vi "Unpack for gRPC.vi"(8 "error in":errorcluster, 9 "configuration / results":enum16{"Configuration", "Results"}(ring), 10 "any":T1, 11 "measurement customizations in":refnum<class "Measurement Plugin.lvclass">) -> (0 "error out":errorcluster, 2 "data value":variant, 3 "measurement customizations out":refnum<class "Measurement Plugin.lvclass">)   [LabVIEW 2024, in "Averaged - Broadband.lvlib" / "Measurement Plugin.lvclass"]
uses:
  Measurement Plugin.lvclass
  <vilib>/gRPC/LabVIEW gRPC Library/Shared/Any.ctl
  Measurement Configuration.ctl
  Measurement Results.ctl
  <vilib>/gRPC/Generated APIs/ni/protobuf/types/RPC Messages/ni_protobuf_types_DoubleXYData.ctl
  a521b266-ce99-437c-923d-067dcf1e07fd.vi
  3ecd018e-d556-4cbc-bc60-c4ba57204520.vi
  <vilib>/gRPC/LabVIEW gRPC Library/Server API/Translate Protobuf Error.vi
  <vilib>/AdvancedString/1D String Array to Delimited String.vi
  <vilib>/gRPC/LabVIEW gRPC Library/Server API/Server/Get Server DLL Path.vi
  Measurement Plugin.lvclass/Measurement Plugin.ctl
  Averaged - Broadband.lvlib
  <vilib>/gRPC/Generated APIs/ni/protobuf/types/ni.protobuf.types.lvlib
  <vilib>/Plug-In SDKs/Measurements/Measurement Plugin Service/Measurement Plugin Service.lvclass
  C:/Program Files/National Instruments/LabVIEW 2024/vi.lib/Plug-In SDKs/Measurements/Measurement Plugin Service/Measurement Plugin Service.lvclass
  C:/Git/dsa/source/FRF Stim-Resp/Averaged - Broadband/Advanced/Measurement Plugin.lvclass
  <vilib>/gRPC/LabVIEW gRPC Library/grpc-lvsupport-release.lvlib
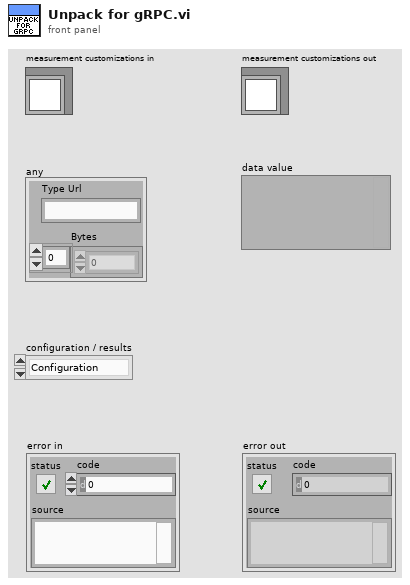
[diagram p1: front panel]
types:
  T1 = typedef "grpc-lvsupport-release.lvlib/Any.ctl" = cluster{"Type Url":string, "Bytes":u8[]}
  T2 = typedef "grpc-lvsupport-release.lvlib/grpcId.ctl" = u64
  T3 = typedef "Averaged - Broadband.lvlib/Measurement Configuration.ctl" = cluster{"double array in":dbl[], "double in":dbl, "U32 array in":u32[], "U32 in":u32, "U64 array in":u64[], "U64 in":u64, "I32 array in":i32[], "I32 in":i32, "I64 array in":i64[], "I64 in":i64, "bool in":bool, "string in":string, "u32 color ring in":u32, "u32 animal enum in":enum32{"Rabbit", "Gopher", "Badger"}}
  T4 = typedef "Averaged - Broadband.lvlib/Measurement Results.ctl" = cluster{"xy data out":T5, "double array out":dbl[], "double out":dbl, "U32 array out":u32[], "U32 out":u32, "U64 array out":u64[], "U64 out":u64, "I32 array out":i32[], "I32 out":i32, "I64 array out":i64[], "I64 out":i64, "bool out":bool, "string out":string, "u32 color ring out":u32, "u32 animal enum out":enum32{"Rabbit", "Gopher", "Badger"}}
  T5 = typedef "ni.protobuf.types.lvlib/ni_protobuf_types_DoubleXYData.ctl" = cluster{"x_data":dbl[], "y_data":dbl[]}
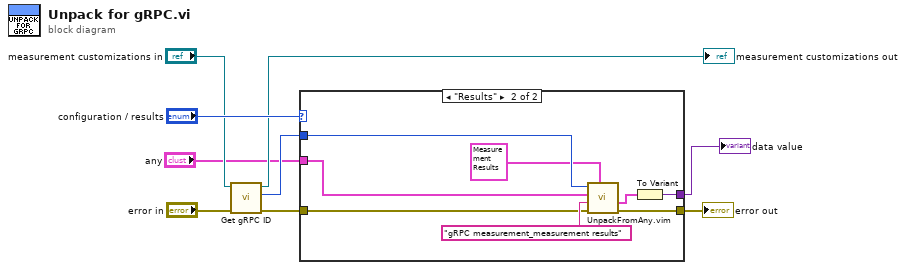
[diagram p0: block diagram]
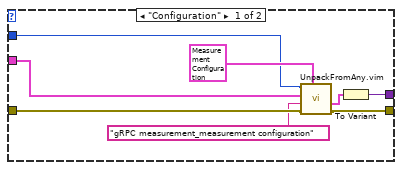
[diagram p2: hidden frame]
diagram:
  n1 = call <vilib>:"Get gRPC ID.vi"("error in"="error in", "measurement plugin service in"="measurement customizations in") -> ("error out"=w6:errorcluster, "gRPC ID"=w3:T2, "measurement plugin service out"=→"measurement customizations out":refnum<class "Measurement Plugin.lvclass">)  [unwired: 7 in]
  n2 = case shown="\"Results\"" "configuration / results" {
    tunnel: w6 -> [w15 w19]
    tunnel: "any" -> [w10 w18]
    tunnel: w3 -> [w12 w22]
    tunnel: [w16 w23] -> w9
    tunnel: [w17 w25] -> w1
    frame "Configuration" {
      n3 = call "UnpackFromAny.vim"("Data Type"=T3 {"double array in"=[], "double in"=1.2, "U32 array in"=[32, 33], "U32 in"=32, "U64 array in"=[64, 65], "U64 in"=64, "I32 array in"=[-32, -33], "I32 in"=-32, "I64 array in"=[-64, -65], "I64 in"=-64, "bool in"=TRUE, "string in"="Lorem ipsum dolor sit", "u32 color ring in"=1, "u32 animal enum in"=enum."Gopher"} ("Measurement Configuration"), "error in"=w15, "Message Type"="gRPC measurement_measurement configuration", "Any"=w10, "gRPCid in"=w12) -> ("error out"=w16:errorcluster, "Unpacked Value"=w14:T3)  [unwired: 4 in, 1 out]
      n4 = To Variant(anything=w14) -> (Variant=w17:variant)
    }
    frame "Results" {
      n5 = call "UnpackFromAny.vim"("Data Type"=T4 {"xy data out"={"x_data"=[], "y_data"=[]}, "double array out"=[], "double out"=0.0, "U32 array out"=[0], "U32 out"=0, "U64 array out"=[0], "U64 out"=0, "I32 array out"=[0], "I32 out"=0, "I64 array out"=[0], "I64 out"=0, "bool out"=FALSE, "string out"="Empty", "u32 color ring out"=0, "u32 animal enum out"=enum."Rabbit"} ("Measurement Results"), "error in"=w19, "Message Type"="gRPC measurement_measurement results", "Any"=w18, "gRPCid in"=w22) -> ("error out"=w23:errorcluster, "Unpacked Value"=w24:T4)  [unwired: 4 in, 1 out]
      n6 = To Variant(anything=w24) -> (Variant=w25:variant)
    }
  }
  "error out" <- w9
  "data value" <- w1
